vi "Set Properties Keithley.vi"(8 "error in (no error)":errorcluster, 11 "Keithley Multimeter in":refnum<class "Keithley Multimeter.lvclass">) -> (0 "error out":errorcluster, 3 "Keithley Multimeter out":refnum<class "Keithley Multimeter.lvclass">)   [LabVIEW 2017, in "Keithley Multimeter.lvclass"]
uses:
  Keithley Multimeter.lvclass
  Keithley Multimeter.lvclass/Keithley Multimeter.ctl
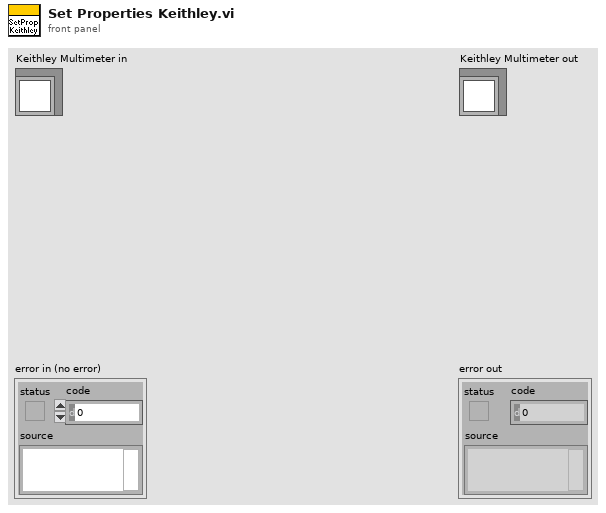
[diagram p1: front panel]
types:
  T1 = cluster{"error":bool, "code":i32, "source":string}
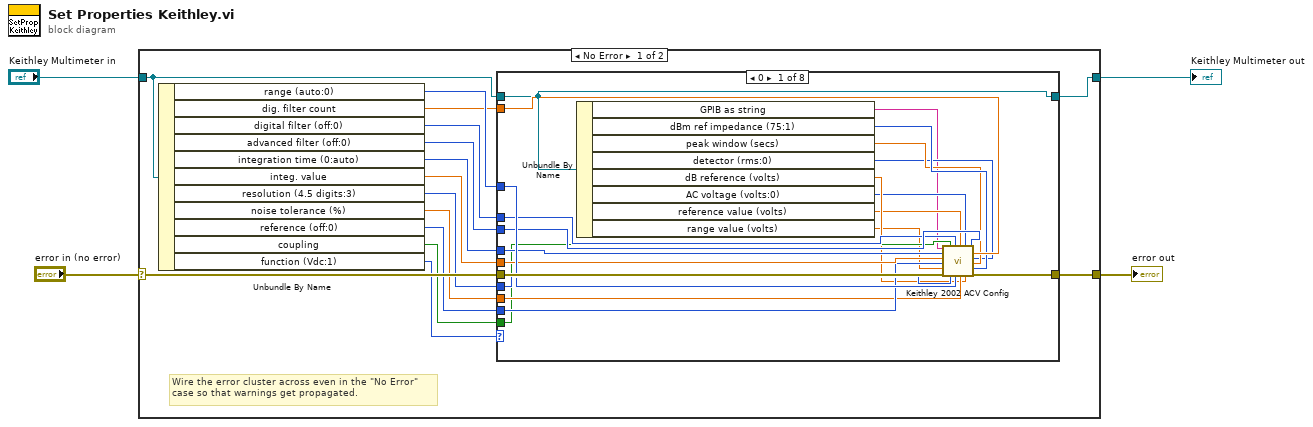
[diagram p0: block diagram]
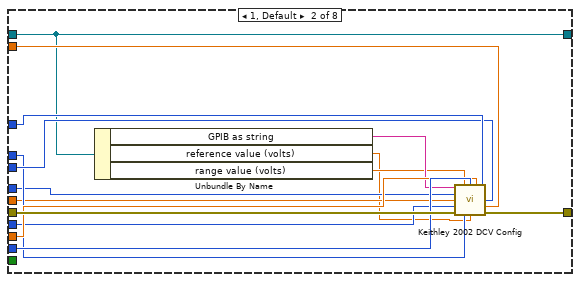
[diagram p2: hidden frame]
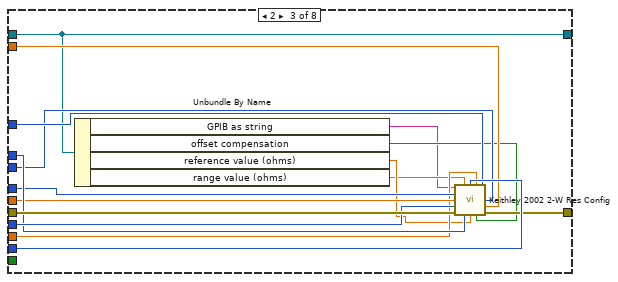
[diagram p3: hidden frame]
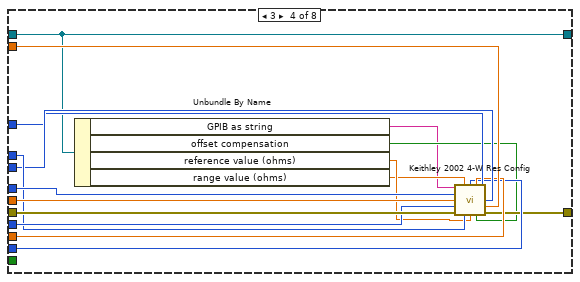
[diagram p4: hidden frame]
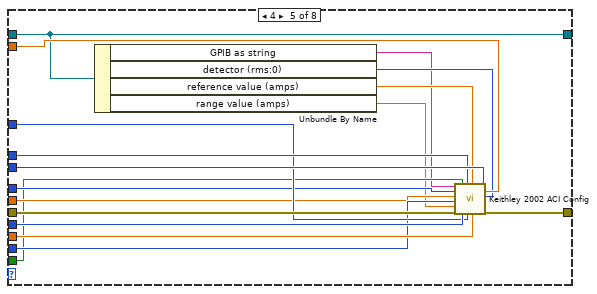
[diagram p5: hidden frame]
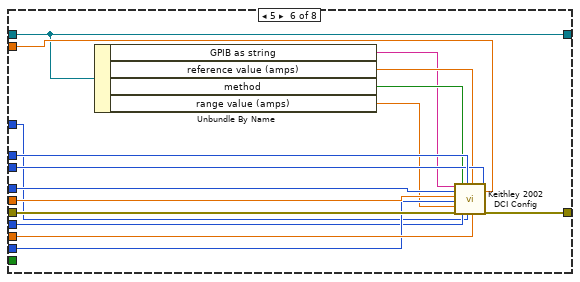
[diagram p6: hidden frame]
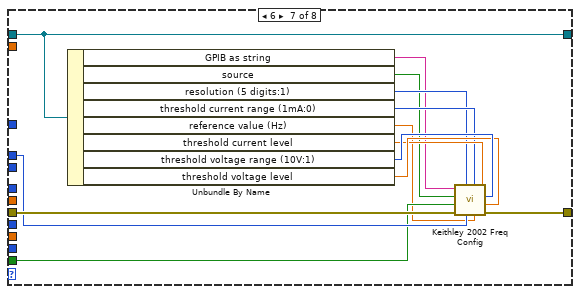
[diagram p7: hidden frame]
diagram:
  n1 = case shown="No Error" "error in (no error)" {
    selector: "error in (no error)" -> [w19 w137]
    tunnel: [w18 w137] -> w3
    tunnel: [w5 w136] -> w1
    tunnel: "Keithley Multimeter in" -> [w6 w136]
    frame No Error {
      # "Wire the error cluster across even in the \"No Error\"\ncase so that warnings get propagated."
      n2 = Unbundle By Name(w6) -> ("range (auto:0)"=w14:u16, "dig. filter count"=w11:dbl, "digital filter (off:0)"=w13:u16, "advanced filter (off:0)"=w16:u16, "integration time (0:auto)"=w12:u16, "integ. value"=w10:dbl, "resolution (4.5 digits:3)"=w9:u16, "noise tolerance (%)"=w17:dbl, "reference (off:0)"=w15:u16, "coupling"=w8:bool, "function (Vdc:1)"=w7:u16)
      n3 = case shown="0" w7 {
        tunnel: w19 -> [w40 w55 w71 w87 w104 w120 w133 w134]
        tunnel: w9 -> [w39 w46 w70 w84 w100 w112 _ _]
        tunnel: w14 -> [w38 w52 w64 w80 w98 w111 _ _]
        tunnel: w11 -> [w32 w50 w62 w82 w103 w119 _ _]
        tunnel: w16 -> [w37 w51 w63 w81 w102 w116 _ _]
        tunnel: w13 -> [w36 w49 w69 w83 w101 w117 w132 _]
        tunnel: w12 -> [w35 w48 w67 w86 w95 w115 _ _]
        tunnel: w10 -> [w34 w47 w68 w85 w96 w114 _ _]
        tunnel: w15 -> [w33 w54 w66 w78 w97 w113 _ _]
        tunnel: w17 -> [w31 w53 w65 w79 w99 w118 _ _]
        tunnel: w8 -> [w30 _ _ _ w94 _ w131 _]
        tunnel: [w29 w45 w61 w77 w93 w110 w130 w134] -> w18
        tunnel: w6 -> [w28 w44 w60 w76 w92 w109 w129 w135]
        tunnel: [w28 w44 w60 w76 w92 w109 w129 w135] -> w5
        frame 0 {
          n4 = Unbundle By Name(w28) -> ("GPIB as string"=w20:string, "dBm ref impedance (75:1)"=w23:u16, "peak window (secs)"=w22:dbl, "detector (rms:0)"=w21:u16, "dB reference (volts)"=w27:dbl, "AC voltage (volts:0)"=w24:u16, "reference value (volts)"=w25:dbl, "range value (volts)"=w26:dbl)
          n5 = call "Keithley 2002 ACV Config.vi"("GPIB address"=w20, "integration time (0:auto)"=w35, "integ. value"=w34, "range (auto:0)"=w33, "range value (volts)"=w26, "error in"=w40, "coupling"=w30, "resolution (4.5 digits:3)"=w39, "reference (off:0)"=w36, "digital filter (off:0)"=w38, "reference value (volts)"=w25, "dig. filter count"=w31, "AC voltage (volts:0)"=w24, "dB reference (volts)"=w27, "advanced filter (off:0)"=w37, "noise tolerance (%)"=w32, "detector (rms:0)"=w21, "peak window (secs)"=w22, "dBm ref impedance (75:1)"=w23) -> ("error out"=w29:T1)
        }
        frame 1, Default {
          n6 = Unbundle By Name(w44) -> ("GPIB as string"=w43:string, "reference value (volts)"=w41:dbl, "range value (volts)"=w42:dbl)
          n7 = call "Keithley 2002 DCV Config.vi"("GPIB address"=w43, "range value (volts)"=w42, "range (auto:0)"=w54, "dig. filter count"=w53, "digital filter (off:0)"=w52, "integration time (0:auto)"=w48, "integ. value"=w47, "advanced filter (off:0)"=w51, "resolution (4.5 digits:3)"=w46, "noise tolerance (%)"=w50, "error in"=w55, "reference (off:0)"=w49, "reference value (volts)"=w41) -> ("error out"=w45:T1)  [unwired: 2 in]
        }
        frame 2 {
          n8 = Unbundle By Name(w60) -> ("GPIB as string"=w56:string, "offset compensation"=w59:bool, "reference value (ohms)"=w58:dbl, "range value (ohms)"=w57:dbl)
          n9 = call "Keithley 2002 2-W Res Config.vi"("GPIB address"=w56, "range value (ohms)"=w57, "range (auto:0)"=w66, "dig. filter count"=w65, "digital filter (off:0)"=w64, "integration time (0:auto)"=w67, "integ. value"=w68, "advanced filter (off:0)"=w63, "resolution (4.5 digits:3)"=w70, "noise tolerance (%)"=w62, "error in"=w71, "reference (off:0)"=w69, "reference value (ohms)"=w58, "offset compensation"=w59) -> ("error out"=w61:T1)  [unwired: 1 in]
        }
        frame 3 {
          n10 = Unbundle By Name(w76) -> ("GPIB as string"=w72:string, "offset compensation"=w75:bool, "reference value (ohms)"=w74:dbl, "range value (ohms)"=w73:dbl)
          n11 = call "Keithley 2002 4-W Res Config.vi"("GPIB address"=w72, "range value (ohms)"=w73, "range (auto:0)"=w78, "dig. filter count"=w79, "digital filter (off:0)"=w80, "integration time (0:auto)"=w86, "integ. value"=w85, "advanced filter (off:0)"=w81, "resolution (4.5 digits:3)"=w84, "noise tolerance (%)"=w82, "error in"=w87, "reference (off:0)"=w83, "reference value (ohms)"=w74, "offset compensation"=w75) -> ("error out"=w77:T1)  [unwired: 1 in]
        }
        frame 4 {
          n12 = Unbundle By Name(w92) -> ("GPIB as string"=w88:string, "detector (rms:0)"=w91:u16, "reference value (amps)"=w90:dbl, "range value (amps)"=w89:dbl)
          n13 = call "Keithley 2002 ACI Config.vi"("GPIB address"=w88, "integration time (0:auto)"=w95, "integ. value"=w96, "range (auto:0)"=w97, "range value (amps)"=w89, "error in"=w104, "coupling"=w94, "resolution (4.5 digits:3)"=w100, "reference (off:0)"=w101, "digital filter (off:0)"=w98, "reference value (amps)"=w90, "dig. filter count"=w99, "advanced filter (off:0)"=w102, "noise tolerance (%)"=w103, "detector (rms:0)"=w91) -> ("error out"=w93:T1)  [unwired: 4 in]
        }
        frame 5 {
          n14 = Unbundle By Name(w109) -> ("GPIB as string"=w105:string, "reference value (amps)"=w108:dbl, "method"=w107:bool, "range value (amps)"=w106:dbl)
          n15 = call "Keithley 2002 DCI Config.vi"("GPIB address"=w105, "integration time (0:auto)"=w115, "integ. value"=w114, "range (auto:0)"=w113, "range value (amps)"=w106, "error in"=w120, "method"=w107, "resolution (4.5 digits:3)"=w112, "reference (off:0)"=w117, "digital filter (off:0)"=w111, "reference value (amps)"=w108, "dig. filter count"=w118, "advanced filter (off:0)"=w116, "noise tolerance (%)"=w119) -> ("error out"=w110:T1)  [unwired: 5 in]
        }
        frame 6 {
          n16 = Unbundle By Name(w129) -> ("GPIB as string"=w121:string, "source"=w123:bool, "resolution (5 digits:1)"=w124:u16, "threshold current range (1mA:0)"=w125:u16, "reference value (Hz)"=w122:dbl, "threshold current level"=w126:dbl, "threshold voltage range (10V:1)"=w128:u16, "threshold voltage level"=w127:dbl)
          n17 = call "Keithley 2002 Freq Config.vi"("threshold voltage level"=w127, "threshold voltage range (10V:1)"=w128, "threshold current level"=w126, "reference value (Hz)"=w122, "threshold current range (1mA:0)"=w125, "reference (off:0)"=w132, "resolution (5 digits:1)"=w124, "error in"=w133, "coupling"=w131, "source"=w123, "GPIB address"=w121) -> ("error out"=w130:T1)
        }
        frame 7 {
        }
      }
    }
    frame Error {
    }
  }
  "error out" <- w3
  "Keithley Multimeter out" <- w1
